vi "Create GrandChildClass.vi"(5 "GrandChildClass in":refnum<class "GrandChildClass.lvclass">, 8 "error in (no error)":errorcluster, 9 "Boolean":bool, 10 "String":string, 11 "Numeric":dbl) -> (0 "error out":errorcluster, 3 "GrandChildClass":refnum<class "GrandChildClass.lvclass">)   [LabVIEW 2017, in "GrandChildClass.lvclass"]
uses:
  GrandChildClass.lvclass
  GrandChildClass.lvclass/GrandChildClass.ctl
  builds/TestLibrary/TestLibrary.lvlibp/Tests/PPL_Inheritance/TestLibrary/ChildClass/ChildClass.lvclass
  C:/Users/pasca/Projects/Home/labview-composition/Tests/PPL_Inheritance/builds/TestLibrary/TestLibrary.lvlibp/Tests/PPL_Inheritance/TestLibrary/ChildClass/ChildClass.lvclass
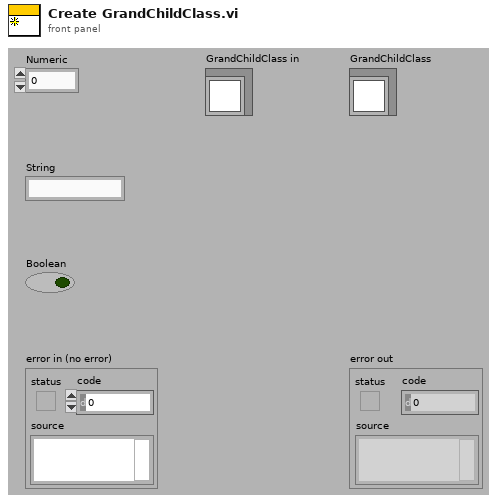
[diagram p1: front panel]
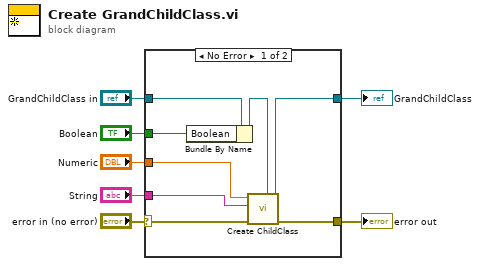
[diagram p0: block diagram]
diagram:
  n1 = case shown="No Error" "error in (no error)" {
    selector: "error in (no error)" -> [w15 w17]
    tunnel: [w12 w17] -> w6
    tunnel: [w13 w16] -> w4
    tunnel: "GrandChildClass in" -> [w14 w16]
    tunnel: "Boolean" -> [w10 _]
    tunnel: "Numeric" -> [w9 _]
    tunnel: "String" -> [w8 _]
    frame No Error {
      n2 = Bundle By Name(cluster=w14, "Boolean"=w10) -> (w11:refnum<class "GrandChildClass.lvclass">)
      n3 = call "Create ChildClass.vi"("ChildClass in"=w11, "error in (no error)"=w15, "String"=w8, "Numeric"=w9) -> ("error out"=w12:errorcluster, "ChildClass"=w13:refnum<class "GrandChildClass.lvclass">)  [unwired: 6 in]
    }
    frame Error {
    }
  }
  "error out" <- w6
  "GrandChildClass" <- w4
